vi "Fitting Configuration 2.vi"() -> (0 "intial guess":dbl[](array[numeric]), 1 "Force Guess？":bool, 2 "Fitting Type":u16(ring) items=["2D Gaussian", "2D Quadrupole", "Double Gaussian", "Double Quadrupole", "Triple Gaussian", "Penta Gaussian"], 3 "Fitting Results Save Path":string[](array[string]))   [LabVIEW 2015]
panel:
  out "Force Guess？ 2":bool
  out "Fitting Type 2":u16(ring) items=["2D Gaussian", "2D Quadrupole", "Double Gaussian", "Double Quadrupole", "Triple Gaussian", "Penta Gaussian"]
  out "Fitting Results Save Path 2":string[](array[string])
  out "intial guess 2":dbl[](array[numeric])
  in  "Force guess？":bool
  in  "Fitting results save path":string[](array[string])
  in  "Component5":dbl[](array[numeric])
  in  "Component4":dbl[](array[numeric])
  in  "Component3":dbl[](array[numeric])
  in  "Component2":dbl[](array[numeric])
  in  "Component1":dbl[](array[numeric])
  in  "Cancel":bool
  in  "OK":bool
  in  "Fitting type":u16(ring) items=["2D Gaussian", "2D Quadrupole", "Double Gaussian", "Double Quadrupole", "Triple Gaussian", "Penta Gaussian"]
  # "1st Component"
  # "2nd Component"
  # "3rd Component"
  # "peak"
  # "xc"
  # "yc"
  # "sigx"
  # "sigy"
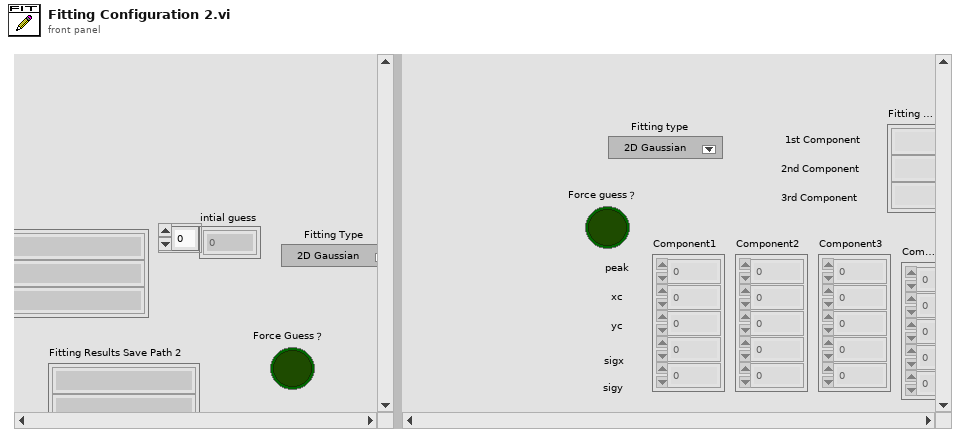
[diagram p1: front panel]
types:
  T1 = enum8{"Enabled", "Disabled", "Disabled and Grayed Out"}
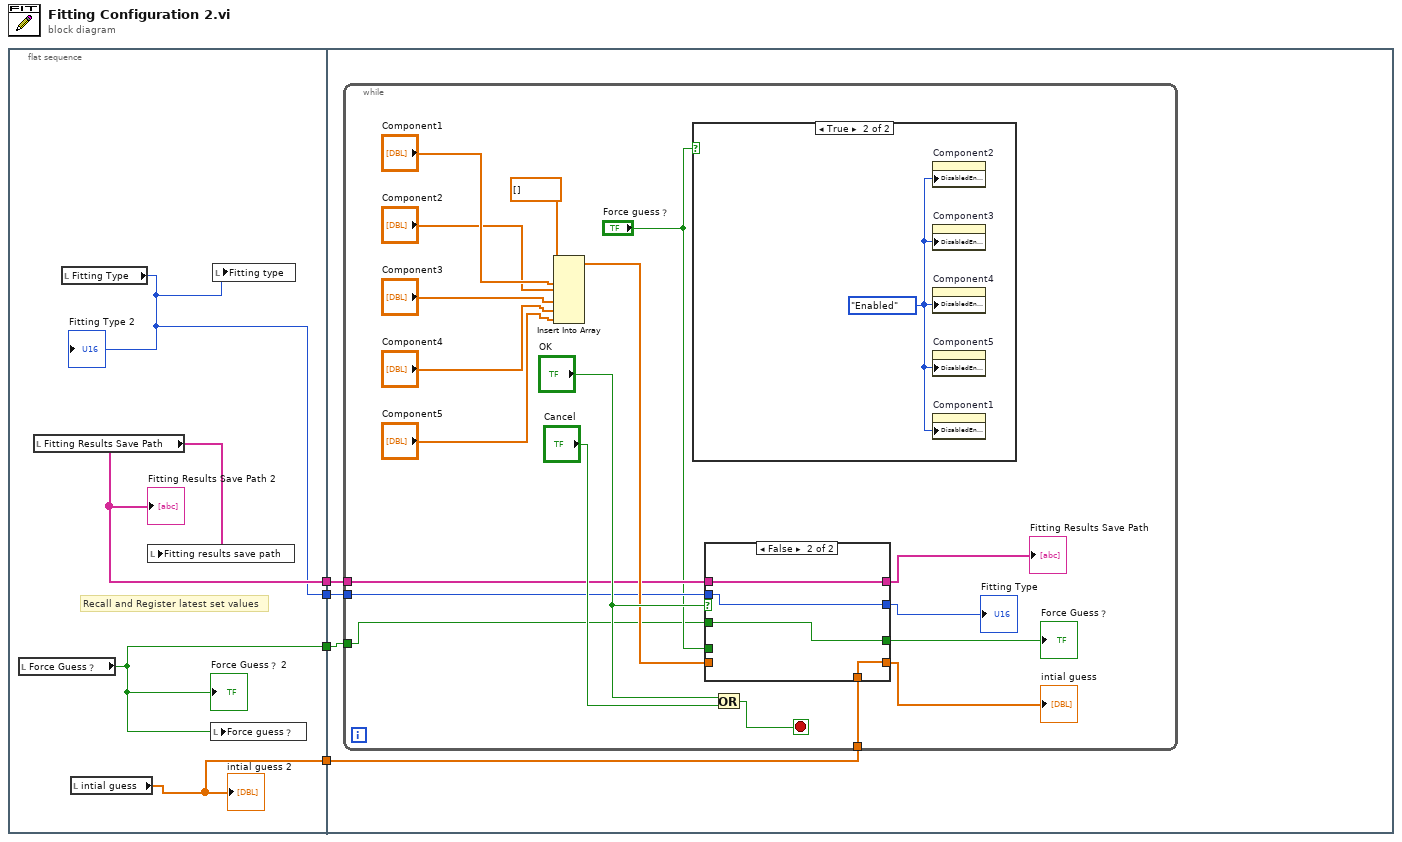
[diagram p0: block diagram]
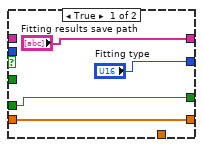
[diagram p2: hidden frame]
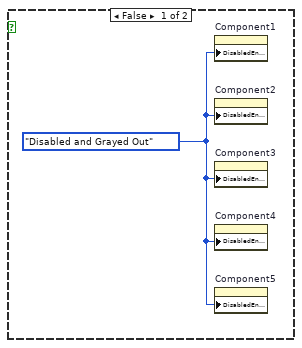
[diagram p3: hidden frame]
diagram:
  n1 = flat-sequence {
    tunnel: [w8] -> w4
    tunnel: [w7] -> w3
    tunnel: [w6] -> w2
    tunnel: [w5] -> w1
    tunnel: w4 -> [w12]
    tunnel: w3 -> [w11]
    tunnel: w2 -> [w10]
    tunnel: w1 -> [w9]
    frame #0 {
      # "Recall and Register latest set values"
      n2 = local read "Force Guess？"() -> (w8:bool)
      "Force Guess？ 2" <- w8
      n3 = local read "Fitting Results Save Path"() -> (w7:string[])
      "Fitting Results Save Path 2" <- w7
      n4 = local read "Fitting Type"() -> (w6:u16)
      "Fitting Type 2" <- w6
      n5 = local read "intial guess"() -> (w5:dbl[])
      "intial guess 2" <- w5
      n6 = local write "Fitting results save path"(w7) -> ()
      n7 = local write "Force guess？"(w8) -> ()
      n8 = local write "Fitting type"(w6) -> ()
    }
    frame #1 {
      n9 = while {
        tunnel: w12 -> [w14]
        tunnel: w11 -> [w17]
        tunnel: w10 -> [w16]
        tunnel: w9 -> [w13]
        stop <- w31 stop-if-true
        n10 = Insert Into Array(array=dbl[] [] ("数组"), new element #1="Component1", new element #2="Component2", new element #3="Component3", new element #4="Component4", new element #5="Component5") -> (w22:dbl[])  [unwired: 1 in]
        n11 = case shown="True" "Force guess？" {
          frame False {
            w40 = T1."Disabled and Grayed Out" ("禁用")
            n12 = property on="Component1" class="Arr (strict)"("DisabledEnum"=w40) -> ()  [unwired: 2 in, 2 out]
            n13 = property on="Component2" class="Arr (strict)"("DisabledEnum"=w40) -> ()  [unwired: 2 in, 2 out]
            n14 = property on="Component3" class="Arr (strict)"("DisabledEnum"=w40) -> ()  [unwired: 2 in, 2 out]
            n15 = property on="Component4" class="Arr (strict)"("DisabledEnum"=w40) -> ()  [unwired: 2 in, 2 out]
            n16 = property on="Component5" class="Arr (strict)"("DisabledEnum"=w40) -> ()  [unwired: 2 in, 2 out]
          }
          frame True {
            w41 = T1."Enabled" ("禁用")
            n17 = property on="Component2" class="Arr (strict)"("DisabledEnum"=w41) -> ()  [unwired: 2 in, 2 out]
            n18 = property on="Component3" class="Arr (strict)"("DisabledEnum"=w41) -> ()  [unwired: 2 in, 2 out]
            n19 = property on="Component4" class="Arr (strict)"("DisabledEnum"=w41) -> ()  [unwired: 2 in, 2 out]
            n20 = property on="Component5" class="Arr (strict)"("DisabledEnum"=w41) -> ()  [unwired: 2 in, 2 out]
            n21 = property on="Component1" class="Arr (strict)"("DisabledEnum"=w41) -> ()  [unwired: 2 in, 2 out]
          }
        }
        n22 = case shown="False" "OK" {
          tunnel: w22 -> [w35 _]
          tunnel: [w35 w36] -> w21
          tunnel: [w32 w37] -> w20
          tunnel: ["Fitting type" w38] -> w19
          tunnel: ["Fitting results save path" w39] -> w18
          tunnel: w17 -> [_ w39]
          tunnel: w16 -> [_ w38]
          tunnel: "Force guess？" -> [w32 _]
          tunnel: w14 -> [_ w37]
          tunnel: w13 -> [_ w36]
          frame True {
          }
          frame False {
          }
        }
        "intial guess" <- w21
        "Force Guess？" <- w20
        "Fitting Type" <- w19
        "Fitting Results Save Path" <- w18
        n23 = Or(x="OK", y="Cancel") -> (x .or. y?=w31:bool)
      }
    }
  }
